vi "CreateVI.vi"(8 "error in (no error)":errorcluster, 9 "Dynamic Dispatch (T)":bool, 10 "Name":string, 11 "CreateClass In":refnum<class "CreateClass.lvclass">) -> (0 "error out":errorcluster, 3 "CreateClass Out":refnum<class "CreateClass.lvclass">)   [LabVIEW 2020, in "Mermaid.lvlib" / "CreateClass.lvclass"]
uses:
  CreateClass.lvclass
  CreateClass.lvclass/CreateClass.ctl
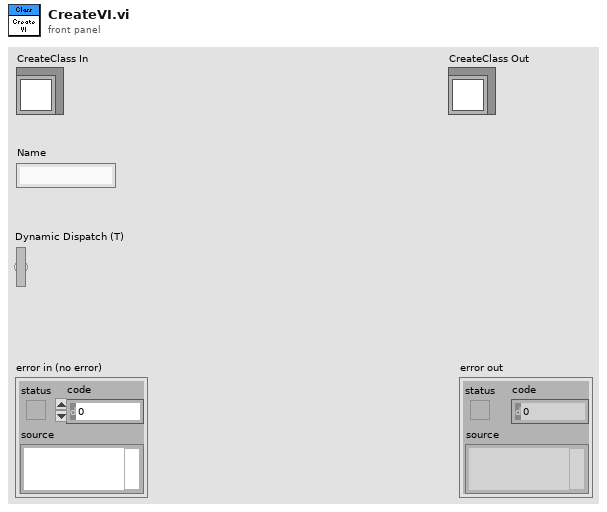
[diagram p1: front panel]
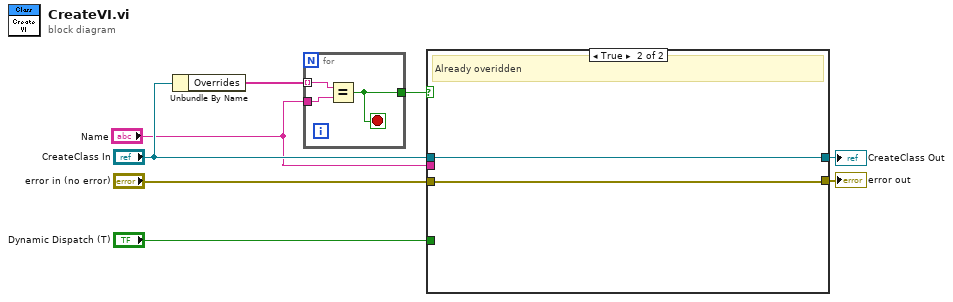
[diagram p0: block diagram]
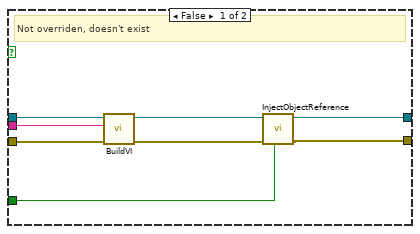
[diagram p2: hidden frame]
diagram:
  n1 = Unbundle By Name("CreateClass In") -> ("Overrides"=w3:string[])
  n2 = for {
    tunnel: w3 -> [w10] mode=indexing
    tunnel: "Name" -> [w11]
    tunnel: [w9] -> w1
    stop <- w9 stop-if-true
    n3 = Equal?(x=w10, y=w11) -> (x = y?=w9:bool)
  }
  n4 = case shown="True" w1 {
    tunnel: "error in (no error)" -> [w19 w20]
    tunnel: [w17 w20] -> w7
    tunnel: [w16 w21] -> w6
    tunnel: "Dynamic Dispatch (T)" -> [w14 _]
    tunnel: "CreateClass In" -> [w13 w21]
    tunnel: "Name" -> [w12 _]
    frame False {
      # "Not overriden, doesn't exist"
      n5 = call "BuildVI.vi"("error in (no error)"=w19, "Name"=w12, "CreateClass In"=w13) -> ("error out"=w18:errorcluster, "CreateClass Out"=w15:refnum<class "CreateClass.lvclass">)  [unwired: 7 in]
      n6 = call "InjectObjectReference.vi"("Dynamic Dispatch"=w14, "error in (no error)"=w18, "CreateClass In"=w15) -> ("error out"=w17:errorcluster, "CreateClass Out"=w16:refnum<class "CreateClass.lvclass">)  [unwired: 7 in]
    }
    frame True {
      # "Already overidden"
    }
  }
  "error out" <- w7
  "CreateClass Out" <- w6
